vi "Grid CellDataWrite.vi"(8 "error in (no error)":errorcluster caption="エラー入力（エラーなし）", 9 "RingText.Text":string, 10 "EditPos":T1, 11 "Table入力":refnum<vi>) -> (0 "エラー出力":errorcluster, 2 "EditPos(copy))":T1 caption="EditPos", 3 "Table出力":refnum<vi>)   [LabVIEW 2014]
uses:
  <vilib>/Utility/miscctls.llb/LVRowAndColumnTypeDef.ctl
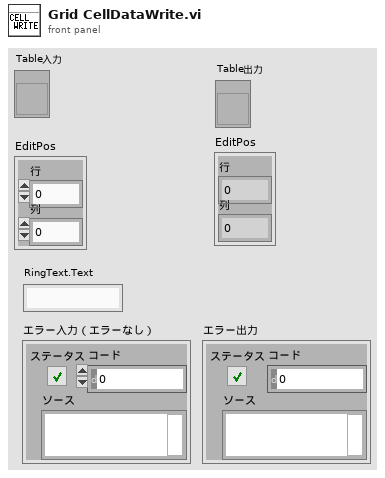
[diagram p1: front panel]
types:
  T1 = typedef "LVRowAndColumnTypeDef.ctl" = cluster{"Row":i32, "Column":i32}
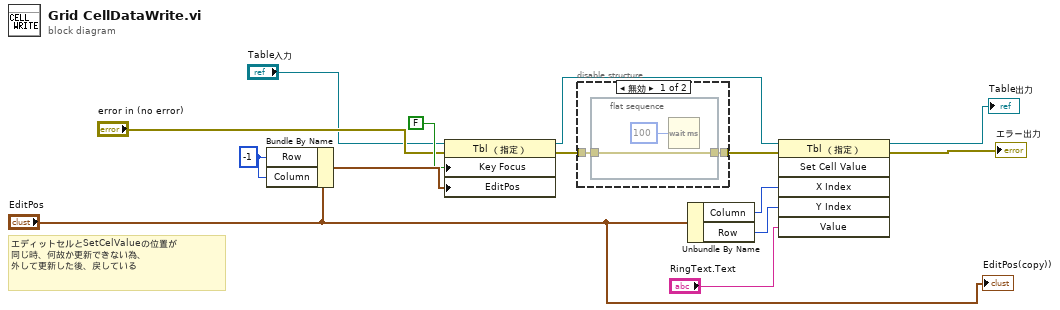
[diagram p0: block diagram]
diagram:
  w5 = -1 ("Row")
  # "エディットセルとSetCelValueの位置が\n同じ時、何故か更新できない為、\n外して更新した後、戻している"
  n1 = Bundle By Name(cluster="EditPos", "Row"=w5, "Column"=w5) -> (w7:T1)
  n2 = property on="プロパティノード" class="Tbl （指定）"(reference="Table入力", error in="error in (no error)", "Key Focus"=FALSE, "EditPos"=w7) -> (reference out=w10:refnum<vi>, error out=w9:errorcluster)
  n3 = disable-structure shown="無効" {
    disable-tunnel: w9 -> [w16 _]
    disable-tunnel: [w15 _] -> w8
    frame Disabled {
      n4 = flat-sequence {
        tunnel: [w18] -> w15
        tunnel: w16 -> [w18]
        frame #0 {
          n5 = Wait (ms)(milliseconds to wait=u32 100 ("ミリ秒待機時間")) -> ()  [unwired: 1 out]
        }
      }
    }
    frame Enabled {
    }
  }
  n6 = Unbundle By Name("EditPos") -> ("Column"=w12:i32, "Row"=w13:i32)
  n7 = invoke on="インボークノード" class="Tbl （指定）" method="Set Cell Value"(reference=w10, error in=w8, "X Index"=w12, "Y Index"=w13, "Value"="RingText.Text") -> (reference out=→"Table出力":refnum<vi>, error out=→"エラー出力":errorcluster)  [unwired: 1 in, 4 out]
  "EditPos(copy))" <- "EditPos"
